vi "HeadPan.vi"(2 "node":string, 3 "error in":errorcluster, 4 "Speed":i32=50, 5 "Units":enum16{"Degrees", "Radians"}(ring), 6 "Pan Angle":sgl) -> (0 "error out":errorcluster)   [LabVIEW 2012]
uses:
  <userlib>/ROSforLV/ROS/Code/Console/Servers/ServerSubs/TopicDef.ctl
  <userlib>/ROSforLV/ROS/Code/SubVIs/_ROSDirection.ctl
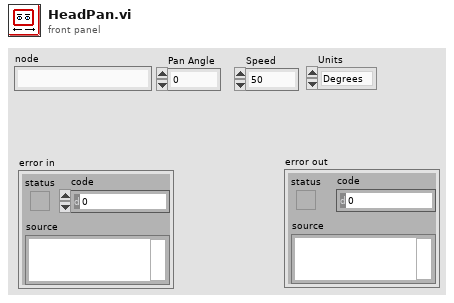
[diagram p1: front panel]
types:
  T1 = typedef "TopicDef.ctl" = cluster{"Topic":string, "Type":string, "Action":T2, "Update (ms)":u16, "write queue":u16}
  T2 = typedef "_ROSDirection.ctl" = enum16{"Node", "Publisher", "Subscriber", "Service Client"}
  T3 = typedef "_ROSControl.ctl" = cluster{"topic port":u16, "Node":string, "topic":string, "type":string, "node port":u32, "error ":errorcluster, "Direction":T2, "APIs":string[], "Update (ms)":u16, "write queue":u16}
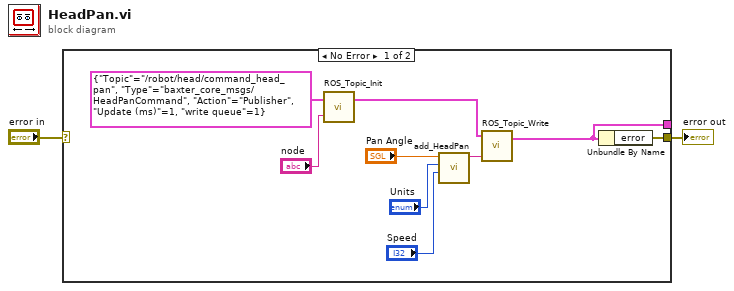
[diagram p0: block diagram]
diagram:
  n1 = case shown="No Error" "error in" {
    selector: "error in" -> [_ w12]
    tunnel: [w10 w12] -> w2
    tunnel: [w8 _] -> _
    frame No Error {
      n2 = call <userlib>:"ROS_Topic_Init.vi"("node"="node", "Definitions"=T1 {"Topic"="/robot/head/command_head_pan", "Type"="baxter_core_msgs/HeadPanCommand", "Action"=enum."Publisher", "Update (ms)"=1, "write queue"=1}) -> ("ROS out"=w11:T3)  [unwired: 1 in]
      n3 = call <userlib>:"add_HeadPan.vi"("Speed"="Speed", "Units"="Units", "Pan Angle"="Pan Angle") -> ("msg out"=w5:string)  [unwired: 8 in]
      n4 = call <userlib>:"ROS_Topic_Write.vi"("Msg in"=w5, "ROS in"=w11) -> ("ROS out"=w8:T3)  [unwired: 2 in]
      n5 = Unbundle By Name(w8) -> ("error"=w10:errorcluster)
    }
    frame Error {
    }
  }
  "error out" <- w2
